vi "Switch Valve.vi"(8 "error in (no error)":errorcluster, 9 "pos":i32, 10 "valve":T1(ring)=enum."BALL_VALVE", 11 "PHD Ultra in":refnum<class "cetoni.lvclass">) -> (0 "error out":errorcluster, 3 "PHD Ultra out":refnum<class "cetoni.lvclass">)   [LabVIEW 2018, in "cetoni.lvlib" / "cetoni.lvclass"]
uses:
  cetoni.lvclass
  <userlib>/QmixLib/QmixLib.lvlib
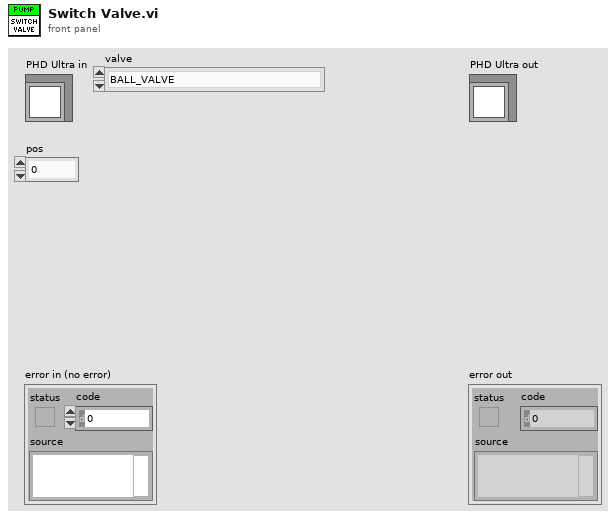
[diagram p1: front panel]
types:
  T1 = enum16{"LOW_PRESSURE_VALVE", "BALL_VALVE", "QMIX_VALVE"}
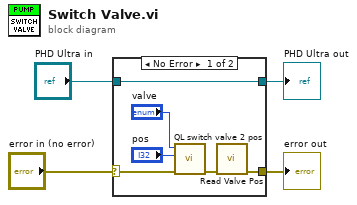
[diagram p0: block diagram]
diagram:
  n1 = case shown="No Error" "error in (no error)" {
    selector: "error in (no error)" -> [w8 w12]
    tunnel: [w5 w12] -> w3
    tunnel: [w10 w11] -> w1
    tunnel: "PHD Ultra in" -> [w10 w11]
    frame No Error {
      n2 = call <userlib>:"QL switch valve 2 pos.vi"("error in (no error)"=w8, "pos"="pos", "valve"="valve") -> ("error out"=w6:errorcluster)  [unwired: 8 in]
      n3 = call "Read Valve Pos.vi"("error in (no error)"=w6) -> ("error out"=w5:errorcluster)  [unwired: 10 in]
    }
    frame Error {
    }
  }
  "error out" <- w3
  "PHD Ultra out" <- w1
